vi "Get Active Worksheet Reference.vi"(8 "error in (no error)":errorcluster, 11 "workbook in":refnum<class "workbook.lvclass">) -> (0 "error out":errorcluster, 2 "Active Worksheet Reference":refnum<k24>, 3 "workbook out":refnum<class "workbook.lvclass">)   [LabVIEW 2017, in "Excel_Specific.lvlib" / "workbook.lvclass"]
uses:
  workbook.lvclass
  C:/Users/Neo/Desktop/Dev_Tools_BR/LabVIEW_NPOI/src/lib/NPOI 2.1.1/NPOI.dll
  lib/NPOI 2.1.1/NPOI.dll
  workbook.lvclass/workbook.ctl
  worksheet/worksheet.lvclass/worksheet.ctl
  worksheet/Get Worksheet.Ref.vi
  worksheet/worksheet.lvclass
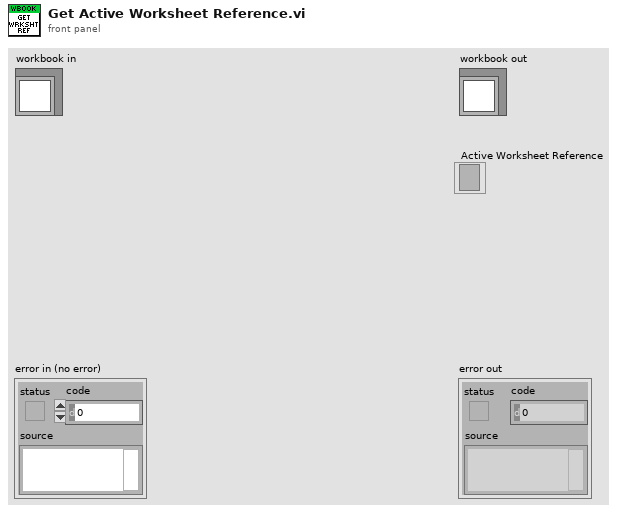
[diagram p1: front panel]
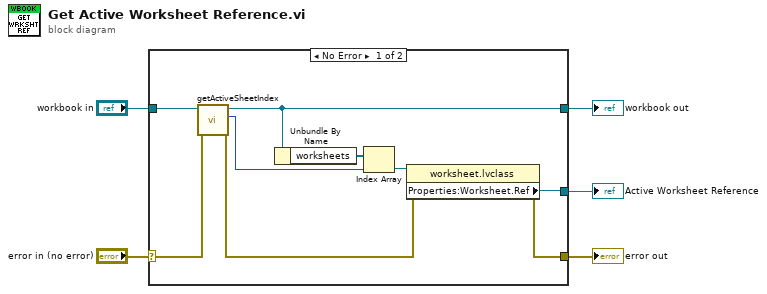
[diagram p0: block diagram]
diagram:
  n1 = case shown="No Error" "error in (no error)" {
    selector: "error in (no error)" -> [w8 w16]
    tunnel: [w11 w16] -> w4
    tunnel: [w9 w15] -> w2
    tunnel: "workbook in" -> [w10 w15]
    tunnel: [w12 _] -> w1
    frame No Error {
      n2 = call "getActiveSheetIndex.vi"("error in (no error)"=w8, "workbook in"=w10) -> ("error out"=w7:errorcluster, "ActiveSheetIndex"=w6:i32, "workbook out"=w9:refnum<class "workbook.lvclass">)  [unwired: 7 in]
      n3 = Unbundle By Name(w9) -> ("worksheets"=w14:refnum<class "worksheet.lvclass">[])
      n4 = Index Array(array=w14, index=w6) -> (element=w13:refnum<class "worksheet.lvclass">)
      n5 = property class="worksheet.lvclass"(reference=w13, error in=w7) -> (error out=w11:errorcluster, "Properties:Worksheet.Ref"=w12:refnum<k24>)  [unwired: 1 out]
    }
    frame Error {
    }
  }
  "error out" <- w4
  "workbook out" <- w2
  "Active Worksheet Reference" <- w1
